vi "File Exist.vi"(2 "File Nm":string, 3 "File path":path) -> (0 "File Exists":bool, 1 "Appended path":path)   [LabVIEW 2016]
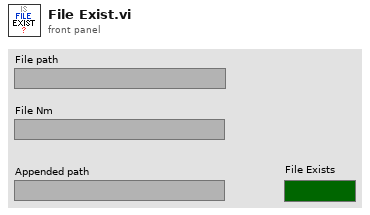
[diagram p1: front panel]
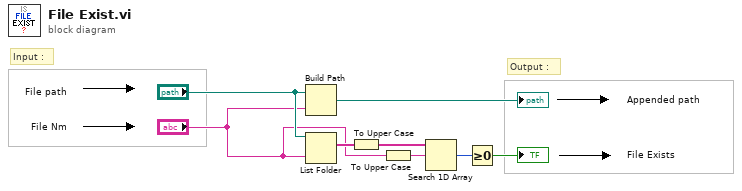
[diagram p0: block diagram]
diagram:
  # "Output :"
  # "Input :"
  n1 = Build Path(base path="File path", name or relative path="File Nm") -> (appended path=→"Appended path":path)
  n2 = List Folder(path="File path", pattern="File Nm") -> (filenames=w6:string[])  [unwired: 2 in, 3 out]
  n3 = To Upper Case(1:w6) -> (0:w2:string[])
  n4 = To Upper Case(1:"File Nm") -> (0:w1:string)
  n5 = Search 1D Array(1D array=w2, element=w1) -> (index of element=w4:i32)  [unwired: 1 in]
  n6 = Greater Or Equal To 0?(x=w4) -> (x >= 0?=→"File Exists":bool)
